vi "PC_CallRTGuidedMunitions.vi"(8 "error in (no error)":errorcluster, 11 "VIParameter":T2={"Machine"="192.168.120.8", "VIPath"=path "C:/ni-rt/startup/Test.vi", "Reentrant?"=FALSE, "InputControlName"="InputControl", "InputControlValue"=variant, "OutputControlName"=""}) -> (0 "error out":errorcluster, 3 "VIOutputParameter":T1={"Machine"="192.168.120.8", "VIPath"=path "C:/ni-rt/startup/Test.vi", "Reentrant?"=FALSE, "InputControlName"="InputControl", "InputControlValue"=variant, "OutputControlName"="", "OutputControlValue"=variant})   [LabVIEW 2010]
uses:
  Ctls/PC_DynCallVIParameter.ctl
  Ctls/PC_DynCallVIOutputParameter.ctl
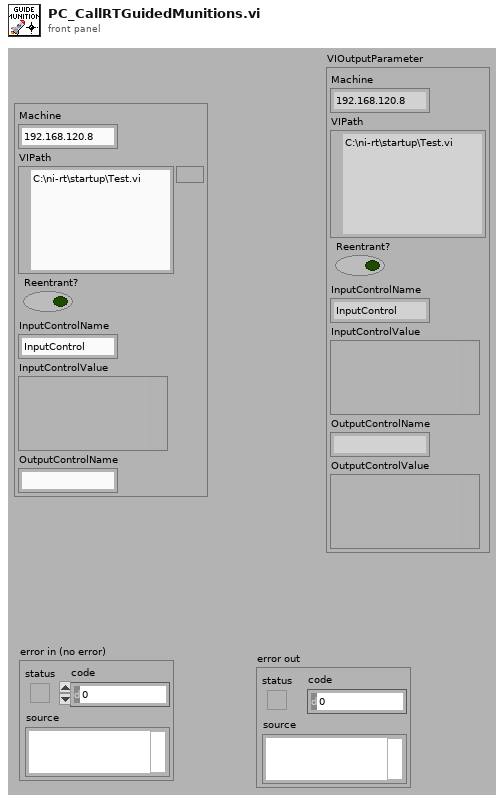
[diagram p1: front panel]
types:
  T1 = typedef "PC_DynCallVIOutputParameter.ctl" = cluster{"Machine":string, "VIPath":path, "Reentrant?":bool, "InputControlName":string, "InputControlValue":variant, "OutputControlName":string, "OutputControlValue":variant}
  T2 = typedef "PC_DynCallVIParameter.ctl" = cluster{"Machine":string, "VIPath":path, "Reentrant?":bool, "InputControlName":string, "InputControlValue":variant, "OutputControlName":string}
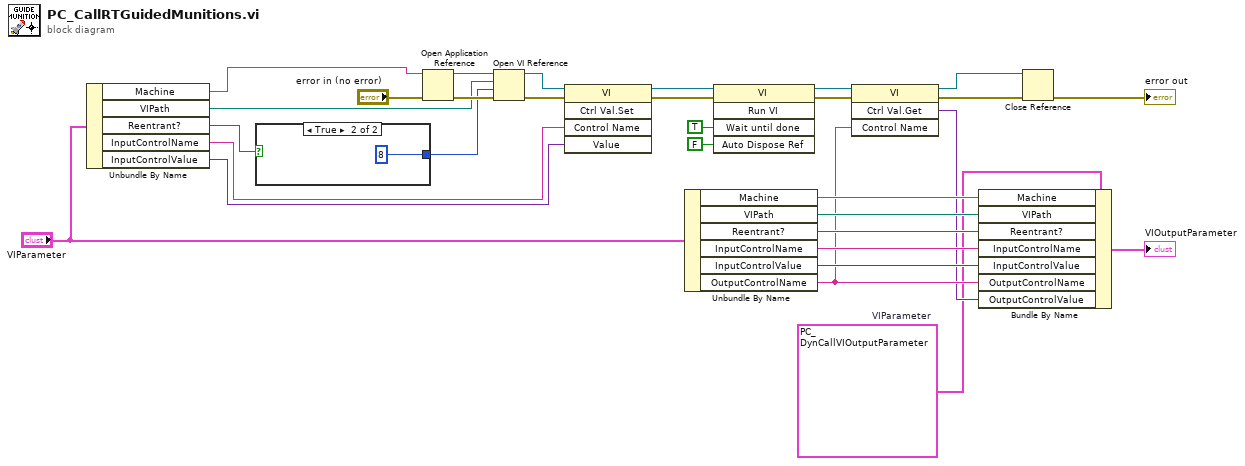
[diagram p0: block diagram]
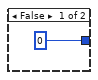
[diagram p2: hidden frame]
diagram:
  w2 = T1 {"Machine"="192.168.120.8", "VIPath"=path "C:/ni-rt/startup/Test.vi", "Reentrant?"=FALSE, "InputControlName"="InputControl", "InputControlValue"=variant, "OutputControlName"="", "OutputControlValue"=variant}  # VIParameter
  n1 = Unbundle By Name("VIParameter") -> ("Machine"=w19:string, "VIPath"=w18:path, "Reentrant?"=w17:bool, "InputControlName"=w16:string, "InputControlValue"=w15:variant)
  n2 = case shown="True" w17 {
    tunnel: [0 ("options") 8 ("options")] -> w24
    frame False {
    }
    frame True {
    }
  }
  n3 = Open Application Reference(8:"error in (no error)", 11:w19) -> (0:w27:errorcluster, 3:w28:refnum<vi>)  [unwired: 2 in]
  n4 = Open VI Reference(application reference (local)=w28, vi path=w18, options=w24, error in (no error)=w27) -> (vi reference=w23:refnum<vi>, error out=w21:errorcluster)  [unwired: 2 in]
  n5 = invoke class="VI" method="Ctrl Val.Set"(reference=w23, error in=w21, "Control Name"=w16, "Value"=w15) -> (reference out=w22:refnum<vi>, error out=w20:errorcluster)  [unwired: 1 in, 3 out]
  n6 = Unbundle By Name("VIParameter") -> ("Machine"=w9:string, "VIPath"=w8:path, "Reentrant?"=w7:bool, "InputControlName"=w6:string, "InputControlValue"=w5:variant, "OutputControlName"=w4:string)
  n7 = invoke class="VI" method="Run VI"(reference=w22, error in=w20, "Wait until done"=TRUE ("Wait Until Done"), "Auto Dispose Ref"=FALSE ("Auto Dispose Reference")) -> (reference out=w14:refnum<vi>, error out=w13:errorcluster)  [unwired: 1 in, 3 out]
  n8 = invoke class="VI" method="Ctrl Val.Get"(reference=w14, error in=w13, "Control Name"=w4) -> (reference out=w11:refnum<vi>, error out=w12:errorcluster, "Get Control Value Variant"=w3:variant)  [unwired: 1 in, 1 out]
  n9 = Bundle By Name(cluster=w2, "Machine"=w9, "VIPath"=w8, "Reentrant?"=w7, "InputControlName"=w6, "InputControlValue"=w5, "OutputControlName"=w4, "OutputControlValue"=w3) -> (→"VIOutputParameter":T1)
  n10 = Close Reference(reference=w11, error in (no error)=w12) -> (error out=→"error out":errorcluster)
